vi "Get Publish Data Events.vi"(11 "UserEvents in":refnum<class "User Events.lvclass">) -> (2 "Publish Data Events":T1, 3 "UserEvents out":refnum<class "User Events.lvclass">)   [LabVIEW 2016, in "User Events.lvclass"]
uses:
  User Events.lvclass
  Typedefs/Publish Data Events.ctl
  Typedefs/StateTypes.ctl
  Typedefs/ScanProgress.ctl
  Typedefs/ActuatorData.ctl
  Typedefs/AllTestStatus.ctl
  Typedefs/TestStatus.ctl
  Typedefs/TestSettings.ctl
  User Events.lvclass/User Events.ctl
  Typedefs/HPMT_Typedefs.lvlib
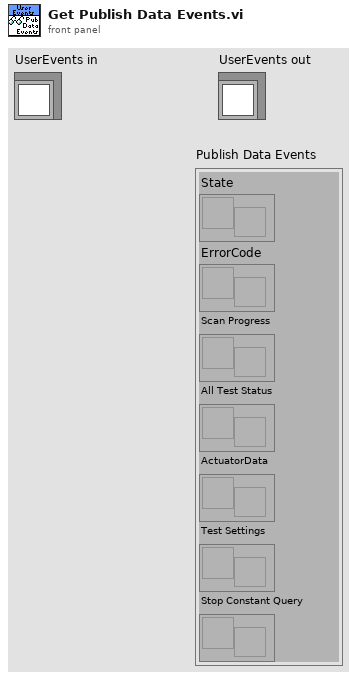
[diagram p1: front panel]
types:
  T1 = typedef "HPMT_Typedefs.lvlib/Publish Data Events.ctl" = cluster{"State":refnum<user-event>, "ErrorCode":refnum<user-event>, "Scan Progress":refnum<user-event>, "All Test Status":refnum<user-event>, "ActuatorData":refnum<user-event>, "Test Settings":refnum<user-event>, "Stop Constant Query":refnum<user-event>}
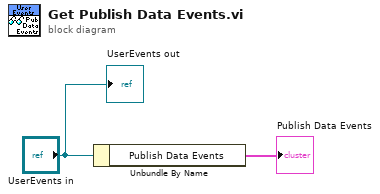
[diagram p0: block diagram]
diagram:
  n1 = Unbundle By Name("UserEvents in") -> ("Publish Data Events"=→"Publish Data Events":T1)
  "UserEvents out" <- "UserEvents in"
